vi "LabviewSPEdatasave_code (not setup).vi"() -> ()   [LabVIEW 2018]
panel:
  in  "Stop After this Acquisition":bool=TRUE
  out "Power vs Gate Delay":cluster{dbl[], dbl[]}(graph)={[740.0, 750.0, 760.0, 770.0, 780.0, 790.0, 800.0, 810.0, 820.0, 830.0, 840.0, 850.0, 860.0], [9735.629577636719, 9727.297424316406, 9722.783203125, 9721.853454589844, 9723.992553710938, 9728.69384765625, 9735.276550292969, 9743.003845214844, 9751.08984375, 9758.719848632812, 9764.941833496094, 9768.833984375, 9769.806823730469]}
  out "Gate delay of peak vs time":dbl[](graph)=[860.0]
  in  "Integration Center WL":dbl=770.0 format="%#_13g"
  in  "WL width":dbl=5.0 format="%#_13g"
  out "Integrated peak vs gate delay":cluster{dbl[], dbl[]}(graph)={[650.0, 700.0, 750.0, 800.0, 850.0, 900.0, 950.0, 1000.0, 1050.0, 1100.0, 1150.0, 1200.0, 1250.0, 1300.0, 1350.0, 1400.0, 1450.0, 1500.0, 1550.0, 1600.0, 1650.0, 1700.0, 1750.0, 1800.0, 1850.0, 1900.0], [368.725, 81.825, 163.675, 339.125, 243.575, 82.55, -16.925, 60.325, 161.775, 63.55, 6.325, 69.075, -40.375, 4.375, 94.0, -26.325, -36.025, -132.65, -113.375, 22.05, -70.375, 7.35, -80.125, 60.75, -80.725, -112.075]}
  out "Spectrum":T1(graph)
  in  "Acuisition type":enum16{"Repetitive", "Sequential"}(ring)=enum."Sequential"
  in  "Acquire":bool
  in  "Gate Start":dbl=650.0 min=1.0 format="%#_13g"
  out "Capture number":i32=3
  out "TDMS error":errorcluster
  out "TDMS file":refnum<k34>
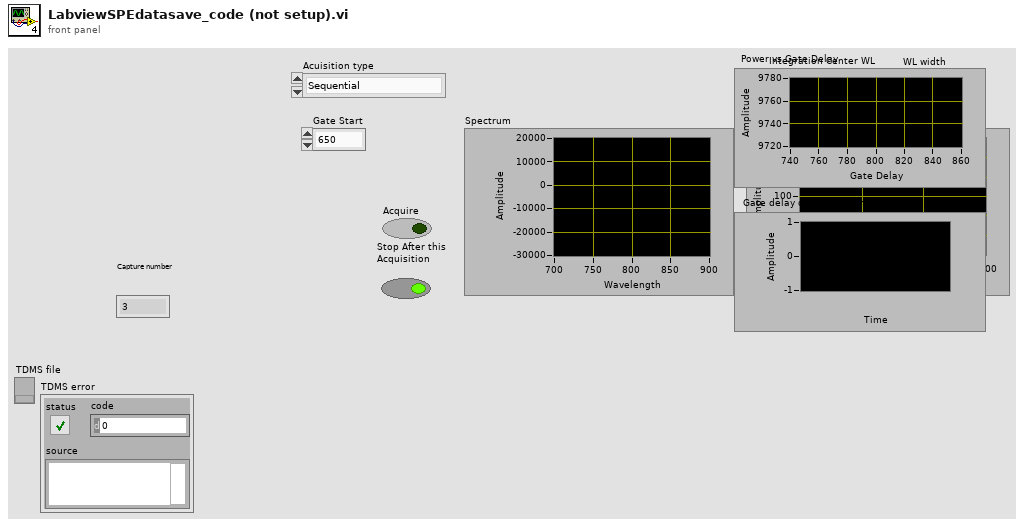
[diagram p1: front panel]
types:
  T1 = cluster{"ColumnCalibration":dbl[], "Image":dbl[]}
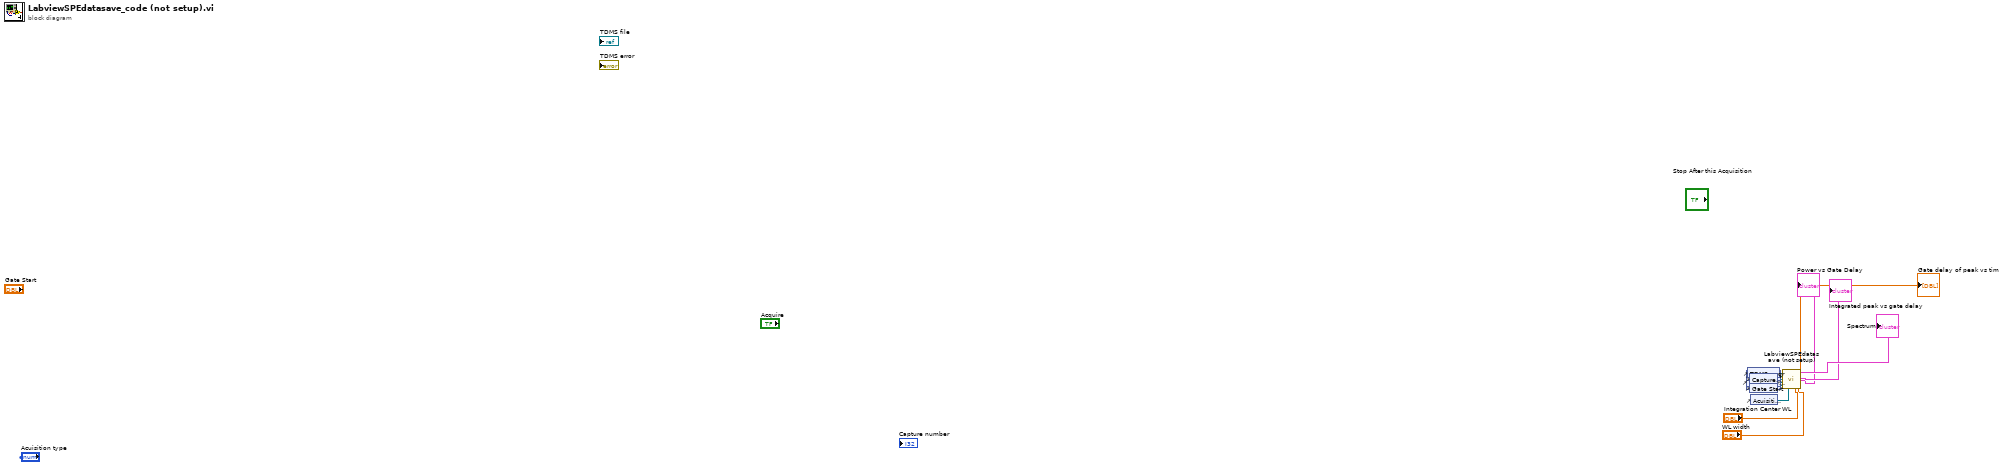
[diagram p0: block diagram]
diagram:
  n1 = control-ref of="TDMS file"() -> (w13:refnum<vi>)
  n2 = control-ref of="Stop After this Acquisition"() -> (w11:refnum<vi>)
  n3 = control-ref of="Acquire"() -> (w10:refnum<vi>)
  n4 = control-ref of="TDMS error"() -> (w14:refnum<vi>)
  n5 = control-ref of="Capture number"() -> (w12:refnum<vi>)
  n6 = control-ref of="Gate Start"() -> (w9:refnum<vi>)
  n7 = control-ref of="Acuisition type"() -> (w8:refnum<vi>)
  n8 = call "LabviewSPEdatasave (not setup).vi"("reference"=w14, "reference 2"=w13, "reference 3"=w12, "reference 4"=w11, "reference 5"=w10, "reference 6"=w9, "reference 7"=w8, "Integration Center WL"="Integration Center WL", "WL width"="WL width") -> ("LightField Automation in"=w16:refnum<class "LightField Automation.lvclass">, "TDMS file"=w18:refnum<k34>, "Camera Setup"=w20:enum16{"Imaging", "Spectral"}, "error in (no error)"=w17:errorcluster, "Gate Width"=w25:dbl, "error in"=w24:errorcluster, "Boolean"=w21:bool, "Image in"=w23:dbl[][][], "New File"=w19:bool, "Save raw Image"=w15:bool, "LightField Automation out"=w27:refnum<class "LightField Automation.lvclass">, "Spectrum"=→"Spectrum":T1, "Image out"=w22:dbl[][][], "Integrated peak vs gate delay"=→"Integrated peak vs gate delay":cluster{dbl[], dbl[]}, "Power vs Gate Delay"=→"Power vs Gate Delay":cluster{dbl[], dbl[]}, "Gate delay of peak vs time"=→"Gate delay of peak vs time":dbl[], "Capture ROI 1, Frame 2"=w1:dbl[][], "error out"=w26:errorcluster)  [unwired: 1 in]
